vi "Remove Headers.vi"(8 "error in (no error)":errorcluster, 11 "HTTP Session in":refnum<class "Session.lvclass">) -> (0 "error out":errorcluster, 3 "HTTP Session out":refnum<class "Session.lvclass">)   [LabVIEW 2015, in "NI_Azure_Core.lvlib" / "Session.lvclass"]
uses:
  Session.lvclass
  Session.lvclass/Session.ctl
  Read HTTP Session.vi
  <vilib>/httpClient/LabVIEWHTTPClient.lvlib
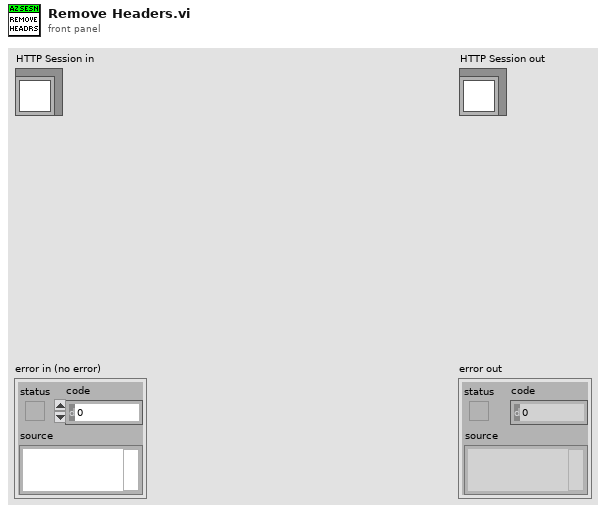
[diagram p1: front panel]
types:
  T1 = typedef "LabVIEWHTTPClient.lvlib/ClientHandle.ctl" = refnum<k1>
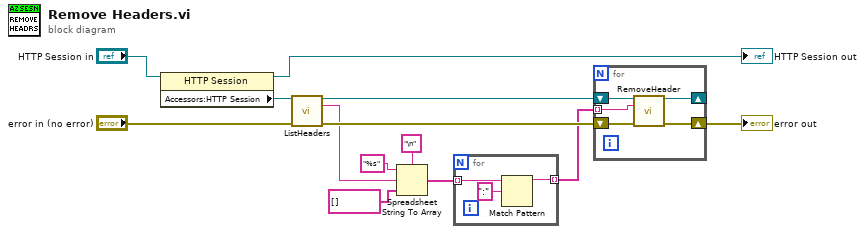
[diagram p0: block diagram]
diagram:
  n1 = property class="HTTP Session"(reference="HTTP Session in") -> (reference out=→"HTTP Session out":refnum<class "Session.lvclass">, "Accessors:HTTP Session"=w3:T1)  [unwired: 1 in, 1 out]
  n2 = call <vilib>:"ListHeaders.vi"("client handle"=w3, "error in (no error)"="error in (no error)") -> ("client handle out"=w13:T1, "headers"=w11:string, "error out"=w12:errorcluster)  [unwired: 11 in]
  n3 = Spreadsheet String To Array(delimiter (Tab)="\n", format string="%s", spreadsheet string=w11, array type (2D Dbl)=string[] []) -> (array=w8:string[])
  n4 = for {
    tunnel: w8 -> [w16] mode=indexing
    tunnel: [w14] -> w6 mode=indexing
    n5 = Match Pattern(string=w16, regular expression=":") -> (before substring=w14:string)  [unwired: 1 in, 3 out]
  }
  n6 = for {
    shift-right: [w18] -> _
    shift-left: w13 -> [w21]
    shift-right: [w19] -> w4
    shift-left: w12 -> [w20]
    tunnel: w6 -> [w17] mode=indexing
    n7 = call <vilib>:"RemoveHeader.vi"("client handle"=w21, "header"=w17, "error in (no error)"=w20) -> ("client handle out"=w18:T1, "error out"=w19:errorcluster)  [unwired: 11 in]
  }
  "error out" <- w4
